vi "Driver Logic Unit.vi"(6 "Ready for Output":bool=TRUE, 7 "Node Number":u8, 8 "error in":errorcluster, 9 "New Cmd Valid?":bool=TRUE, 10 "Command sent by Node":T3, 11 "Private Data In":T2={"DLU To SPI Engine Data FIFO"="DLU To SPI Engine Data", "SPI Engine to DLU Data FIFO"="SPI Engine to DLU Data", "Data to SPI Engine (Cache) Register"="Data to SPI Engine (Cache)", "SPI PHY Settings to SPI Engine (Cahche) Register"="SPI PHY Settings to SPI Engine (Cache)"}) -> (0 "error out":errorcluster, 1 "SPI Data Valid?":bool, 2 "SPI Bus Read Data":T1, 4 "Ready For Input?":bool)   [LabVIEW 2014, in "IO Node Logic Template_SPIBus1.lvlib"]
uses:
  IO Node Logic Template_SPIBus1.lvlib
  IONode/Node/Controls/Node_Command_Sent.ctl
  <vilib>/SPI API/SPIAPI/Controls/Internal Data (SPI API).ctl
  <vilib>/SPI API/SPIAPI/Controls/SPI Response Information.ctl
  Controls/Driver Logic Unit State.ctl
  <userlib>/_NI SPI IP/FPGA/Controllers/Public/Transfer Settings.ctl
  <userlib>/_NI SPI IP/FPGA/Controllers/NI SPI IP FPGA.lvlib
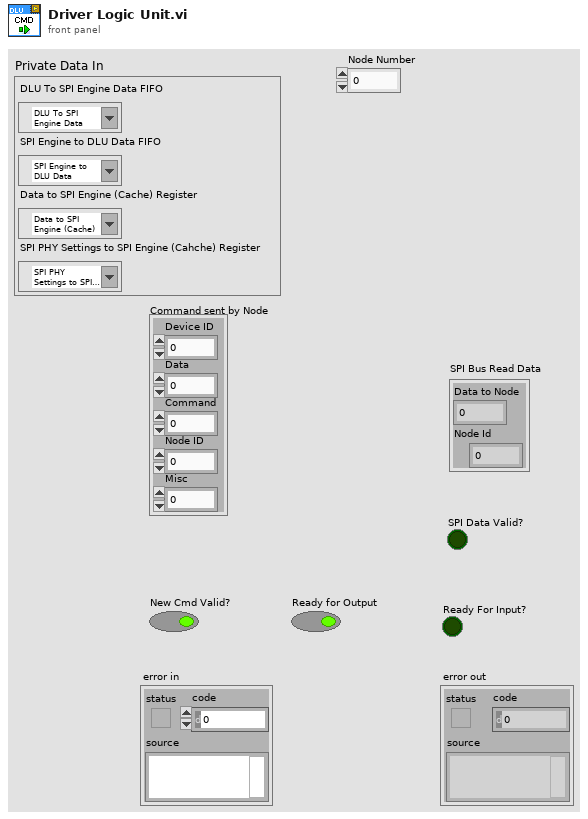
[diagram p1: front panel]
types:
  T1 = typedef "SPI Response Information.ctl" = cluster{"Data to Node":u64, "Node Id":u16}
  T2 = typedef "Internal Data (SPI API).ctl" = cluster{"DLU To SPI Engine Data FIFO":refnum<k21>, "SPI Engine to DLU Data FIFO":refnum<k21>, "Data to SPI Engine (Cache) Register":refnum<k21>, "SPI PHY Settings to SPI Engine (Cahche) Register":refnum<k21>}
  T3 = typedef "Node_Command_Sent.ctl" = cluster{"Device ID":u8, "Data":u64, "Command":u8, "Node ID":u8, "Misc":u8}
  T4 = typedef "NI SPI IP FPGA.lvlib/Transfer Settings.ctl" = cluster{"Divide Value":u8, "Transfer Length (bits)":u8, "CS Asserted Polarity":bool, "Clock Polarity (CPOL)":bool, "Clock Phase (CPHA)":bool, "Lengthen MISO Setup":bool, "Direction Change Bit":u8, "MOSI Starts as Output":bool, "Tristatable MOSI":bool}
  T5 = typedef "IO Node Logic Template_SPIBus1.lvlib/Driver Logic Unit State.ctl" = enum16{"Idle", "Sequence1: Start", "Sequence1: Step1", "Sequence1: Step2", "Sequence1: Step3", "Sequence1: Step4", "Sequence1: End"}
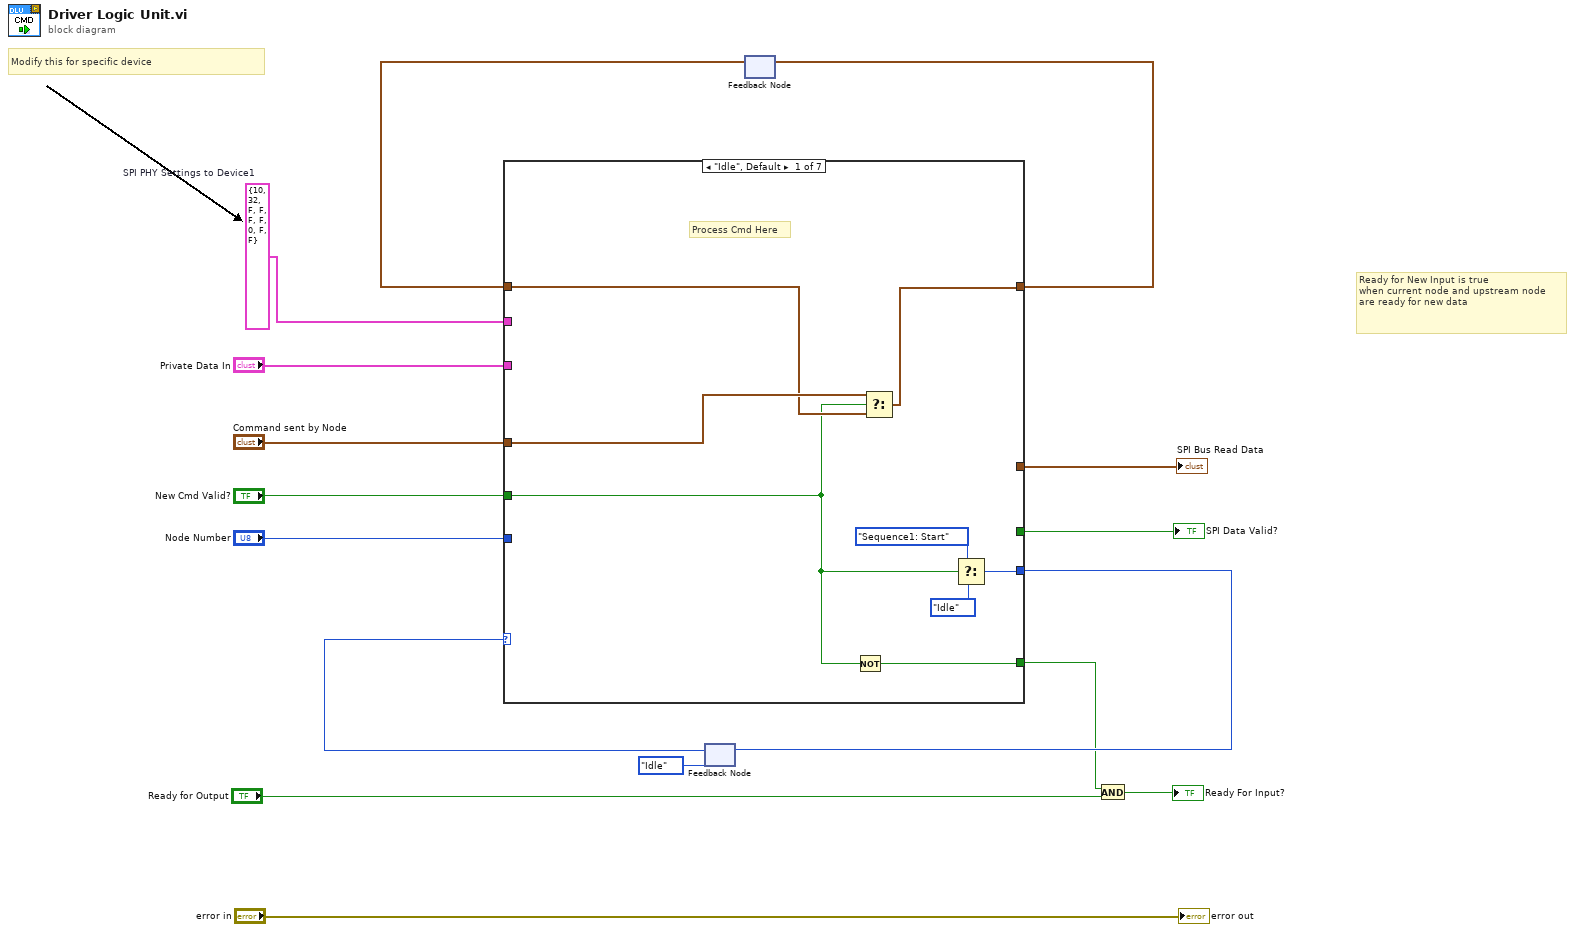
[diagram p0: block diagram]
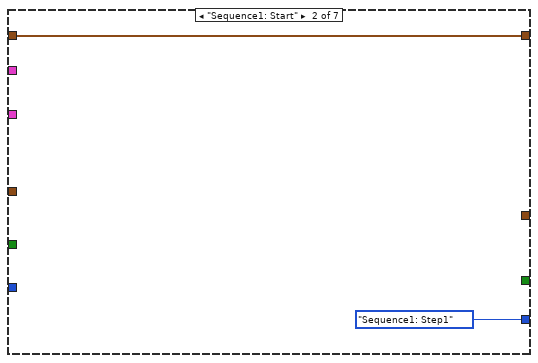
[diagram p2: hidden frame]
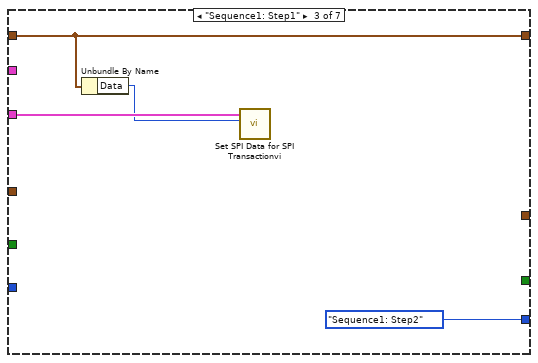
[diagram p3: hidden frame]
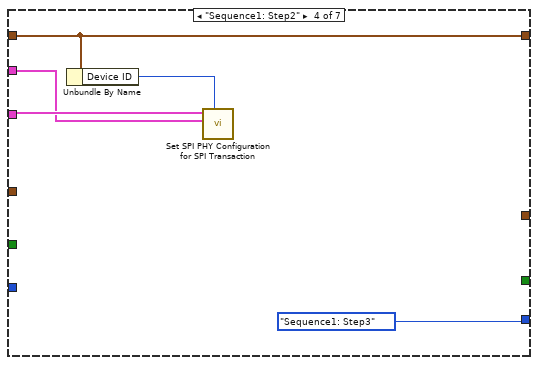
[diagram p4: hidden frame]
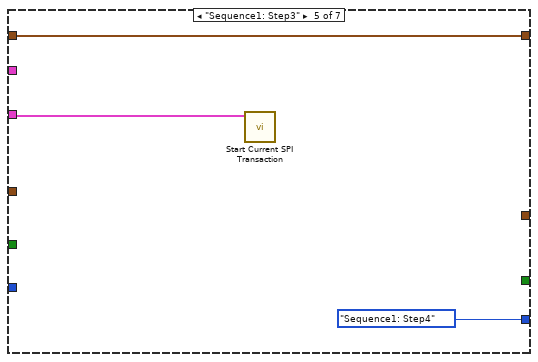
[diagram p5: hidden frame]
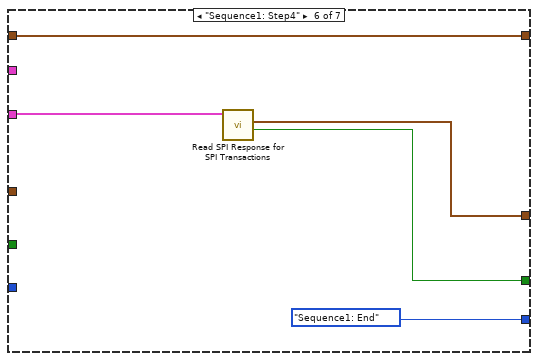
[diagram p6: hidden frame]
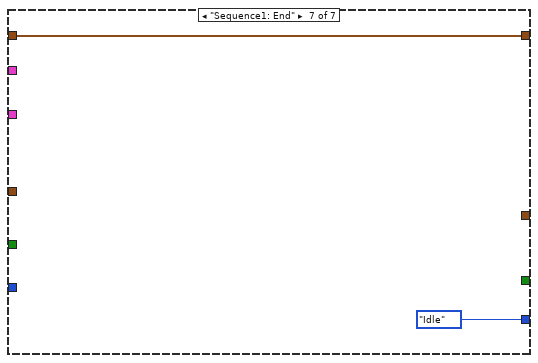
[diagram p7: hidden frame]
diagram:
  w1 = T4 {"Divide Value"=10, "Transfer Length (bits)"=32, "CS Asserted Polarity"=FALSE, "Clock Polarity (CPOL)"=FALSE, "Clock Phase (CPHA)"=FALSE, "Lengthen MISO Setup"=FALSE, "Direction Change Bit"=0, "MOSI Starts as Output"=FALSE, "Tristatable MOSI"=FALSE}  # SPI PHY Settings to Device1
  # "Modify this for specific device"
  # "Ready for New Input is true\nwhen current node and upstream node\nare ready for new data"
  n1 = feedback #1(Driver_Logic_Unit_State."Idle") -> (w15:T5)
  n2 = feedback #2() -> (w2:T3)  [unwired: 1 in]
  n3 = case shown="\"Idle\", Default" w15 {
    tunnel: [w21 _ _ _ _ _ _] -> w8
    tunnel: [w23 Driver_Logic_Unit_State."Sequence1: Step1" Driver_Logic_Unit_State."Sequence1: Step2" Driver_Logic_Unit_State."Sequence1: Step3" Driver_Logic_Unit_State."Sequence1: Step4" Driver_Logic_Unit_State."Sequence1: End" Driver_Logic_Unit_State."Idle"] -> w16
    tunnel: "New Cmd Valid?" -> [w17 _ _ _ _ _ _]
    tunnel: "Command sent by Node" -> [w20 _ _ _ _ _ _]
    tunnel: [_ _ _ _ _ w43 _] -> w13
    tunnel: [_ _ _ _ _ w42 _] -> w4
    tunnel: "Node Number" -> [_ _ _ _ _ _ _]
    tunnel: "Private Data In" -> [_ _ w30 w35 w37 w40 _]
    tunnel: w2 -> [w18 w25 w27 w32 w36 w39 w44]
    tunnel: [w19 w25 w27 w32 w36 w39 w44] -> w3
    tunnel: w1 -> [_ _ _ w33 _ _ _]
    frame "Idle", Default {
      # "Process Cmd Here"
      n4 = Not(x=w17) -> (.not. x?=w21:bool)
      n5 = Select(t=w20, s=w17, f=w18) -> (s? t:f=w19:T3)
      n6 = Select(t=Driver_Logic_Unit_State."Sequence1: Start", s=w17, f=Driver_Logic_Unit_State."Idle") -> (s? t:f=w23:T5)
    }
    frame "Sequence1: Start" {
    }
    frame "Sequence1: Step1" {
      n7 = Unbundle By Name(w27) -> ("Data"=w28:u64)
      n8 = call <vilib>:"Set SPI Data for SPI Transactionvi.vi"("Data In"=w28, "Private Data In"=w30) -> ()  [unwired: 8 in, 2 out]
    }
    frame "Sequence1: Step2" {
      n9 = Unbundle By Name(w32) -> ("Device ID"=w31:u8)
      n10 = call <vilib>:"Set SPI PHY Configuration for SPI Transaction.vi"("Chip Select"=w31, "SPI PHY Settings"=w33, "Private Data In"=w35) -> ()  [unwired: 7 in, 2 out]
    }
    frame "Sequence1: Step3" {
      n11 = call <vilib>:"Start Current SPI Transaction.vi"("Private Data In"=w37) -> ()  [unwired: 8 in, 3 out]
    }
    frame "Sequence1: Step4" {
      n12 = call <vilib>:"Read SPI Response for SPI Transactions.vi"("Private Data In"=w40) -> ("Read Data Valid?"=w43:bool, "Read Data"=w42:T1)  [unwired: 7 in, 2 out]
    }
    frame "Sequence1: End" {
    }
  }
  "SPI Data Valid?" <- w13
  "SPI Bus Read Data" <- w4
  n13 = feedback-in #1(w16) -> ()
  n14 = feedback-in #2(w3) -> ()
  n15 = And(x=w8, y="Ready for Output") -> (x .and. y?=→"Ready For Input?":bool)
  "error out" <- "error in"
